vi "outDictSel.vi"(8 "error in (no error)":errorcluster, 10 "On/Off Data":bool, 11 "Select Macro Function":T1(radio)) -> (0 "error out":errorcluster, 3 "Dictionary Selector":string)   [LabVIEW 2019]
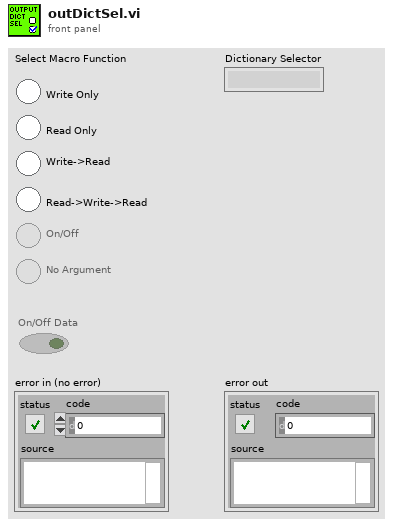
[diagram p1: front panel]
types:
  T1 = enum32{"No Selection", "WRITE", "READ", "WRITE -> READ", "READ -> WRITE -> READ", "ON/OFF", "NO ARGS"}
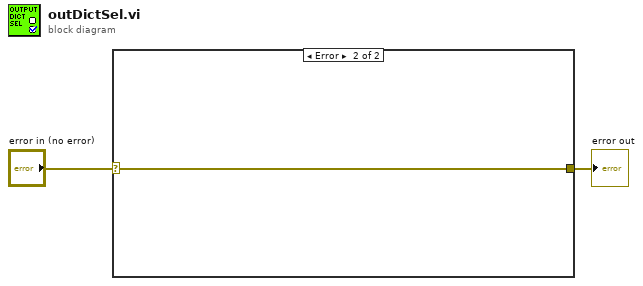
[diagram p0: block diagram]
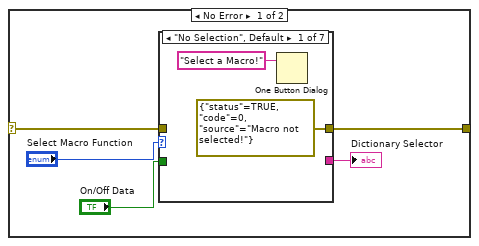
[diagram p2: hidden frame]
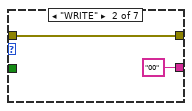
[diagram p3: hidden frame]
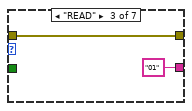
[diagram p4: hidden frame]
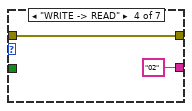
[diagram p5: hidden frame]
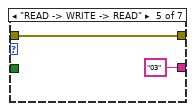
[diagram p6: hidden frame]
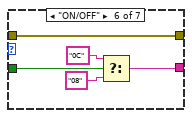
[diagram p7: hidden frame]
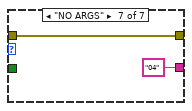
[diagram p8: hidden frame]
diagram:
  n1 = case shown="Error" "error in (no error)" {
    selector: "error in (no error)" -> [w3 w25]
    tunnel: [w6 w25] -> w2
    frame No Error {
      n2 = case shown="\"No Selection\", Default" "Select Macro Function" {
        tunnel: [_ "00" "01" "02" "03" w20 "04"] -> w7
        tunnel: "On/Off Data" -> [_ _ _ _ _ w19 _]
        tunnel: w3 -> [_ w10 w12 w14 w16 w18 w23]
        tunnel: [errorcluster {"status"=TRUE, "code"=0, "source"="Macro not selected!"} ("error constant") w10 w12 w14 w16 w18 w23] -> w6
        frame "No Selection", Default {
          n3 = One Button Dialog(message="Select a Macro!") -> ()  [unwired: 1 in, 1 out]
        }
        frame "WRITE" {
        }
        frame "READ" {
        }
        frame "WRITE -> READ" {
        }
        frame "READ -> WRITE -> READ" {
        }
        frame "ON/OFF" {
          n4 = Select(t="0C", s=w19, f="08") -> (s? t:f=w20:string)
        }
        frame "NO ARGS" {
        }
      }
      "Dictionary Selector" <- w7
    }
    frame Error {
    }
  }
  "error out" <- w2
